vi "Create.vi"(8 "error in (no error)":errorcluster, 10 "EnQr":refnum<class "Message Enqueuer.lvclass">) -> (0 "error out":errorcluster, 3 "AbortAPI out":refnum<class "AbortAPI.lvclass">)   [LabVIEW 2020, in "Volatus.lvlib" / "AbortAPI.lvclass"]
uses:
  AbortAPI.lvclass
  AbortAPI.lvclass/AbortAPI.ctl
  <vilib>/ActorFramework/Message Enqueuer/Message Enqueuer.lvclass
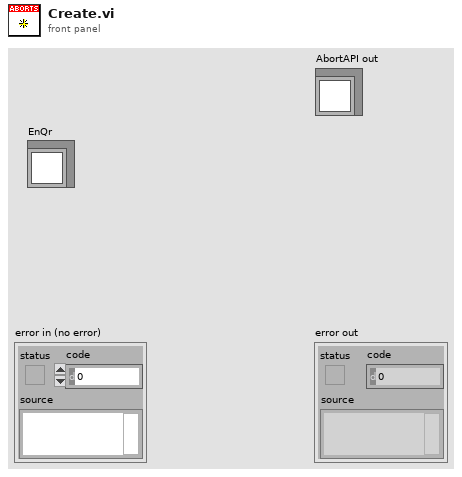
[diagram p1: front panel]
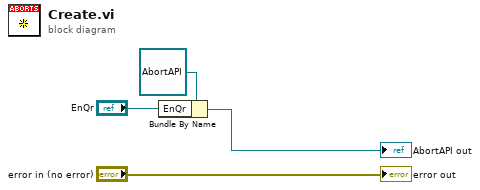
[diagram p0: block diagram]
diagram:
  n1 = Bundle By Name(cluster=refnum<class "AbortAPI.lvclass"> refnum ("AbortAPI in"), "EnQr"="EnQr") -> (→"AbortAPI out":refnum<class "AbortAPI.lvclass">)
  "error out" <- "error in (no error)"
